vi "tsapp_add_cyclic_msg_can_win32.vi"(8 "错误输入（无错误）":errorcluster, 9 "AAppChannel":i32(ring) items=["CHN1", "CHN2", "CHN3", "CHN4", "CHN5", "CHN6", "CHN7", "CHN8", "CHN9", "CHN10", "CHN11", "CHN12", "CHN13", "CHN14", "CHN15", "CHN16", "CHN17", "CHN18", "CHN19", "CHN20", "CHN21", "CHN22", "CHN23", "CHN24", "CHN25", "CHN26", "CHN27", "CHN28", "CHN29", "CHN30", "CHN31", "CHN32"], 10 "APeriodMS":sgl, 11 "数据帧信息":T1 {"ADLC" max=64; "AID" max=536870911}) -> (0 "错误输出":errorcluster, 3 "tsapp_add_cyclic_msg_can":i32)   [LabVIEW 2016]
uses:
  Ctrl/CAN_FrameInfo.ctl
  TCANProperty.ctl
  SendMsgInfo.ctl
  TSMaster.dll
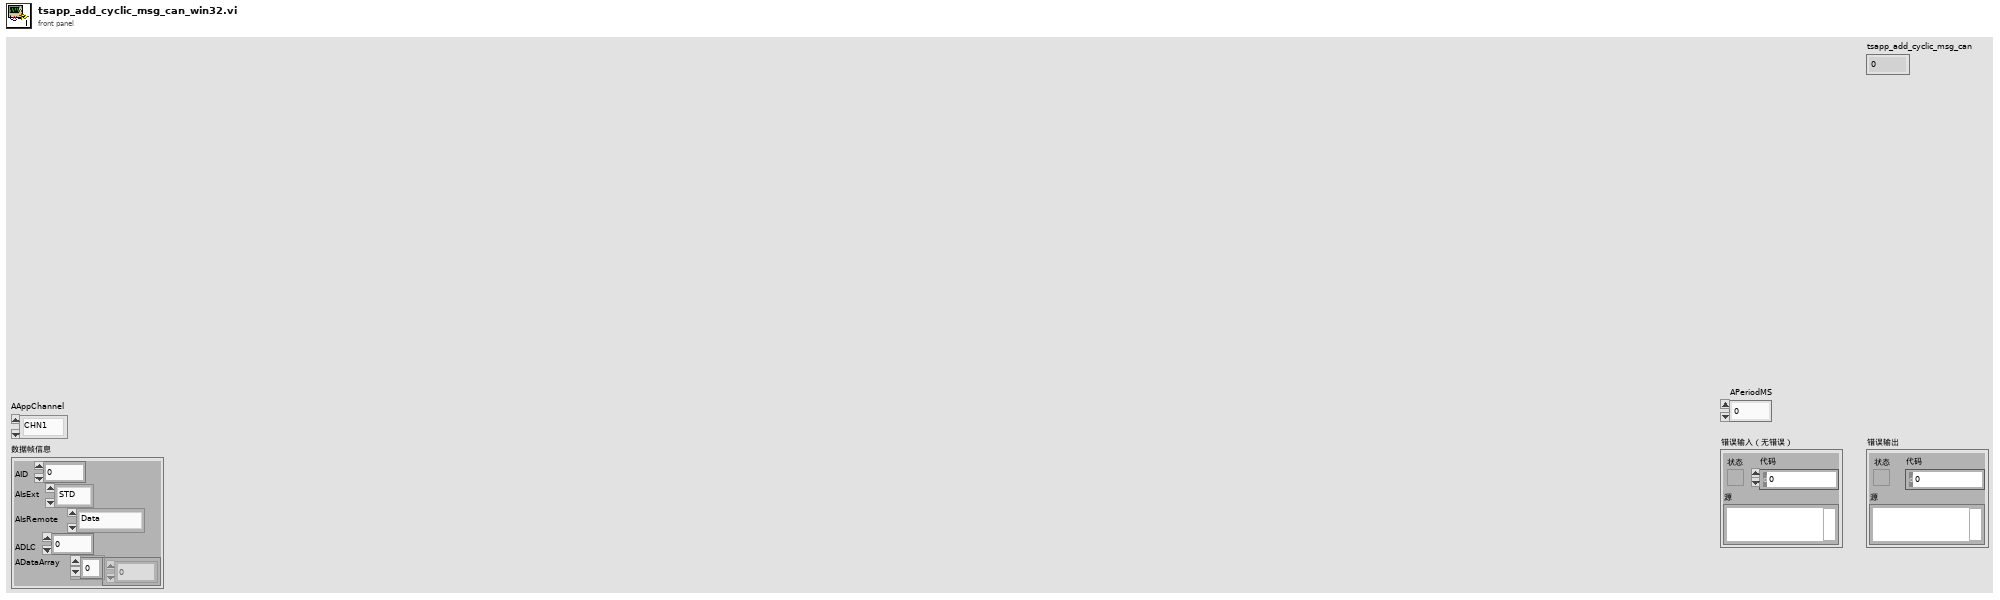
[diagram p1: front panel]
types:
  T1 = typedef "CAN_FrameInfo.ctl" = cluster{"AID":u32, "AIsExt":enum16{"STD", "EXT"}, "AIsRemote":enum16{"Data", "Remote"}, "ADLC":u8, "ADataArray":u8[]}
  T2 = typedef "SendMsgInfo.ctl" = cluster{"FIdxChn":u8, "FProperties":u8, "FDLC":u8, "FReserved":u8, "FIdentifier":i32, "FTimeUS":u64, "Data0":u8, "Data1":u8, "Data2":u8, "Data3":u8, "Data4":u8, "Data5":u8, "Data6":u8, "Data7":u8}
  T3 = typedef "TCANProperty.ctl" = cluster{"istx":bool, "remoteframe":bool, "extframe":bool, "tbd1":bool, "tbd2":bool, "tbd3":bool, "tbd4":bool, "iserrorframe":bool}
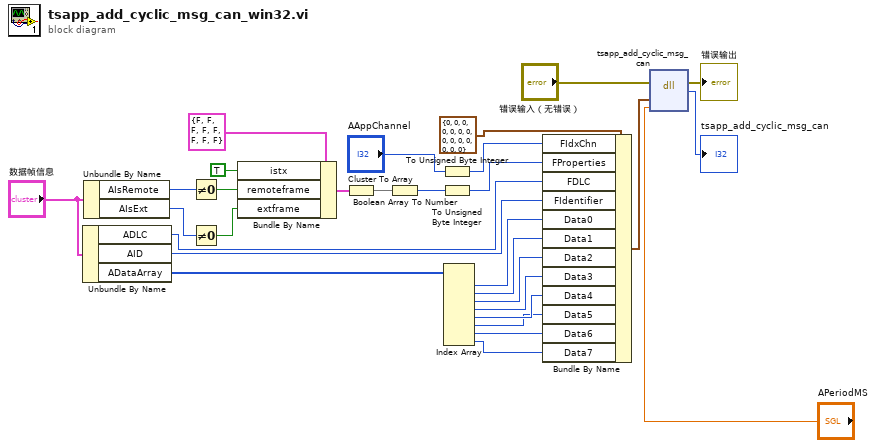
[diagram p0: block diagram]
diagram:
  n1 = Unbundle By Name("数据帧信息") -> ("ADLC"=w12:u8, "AID"=w11:u32, "ADataArray"=w10:u8[])
  n2 = Unbundle By Name("数据帧信息") -> ("AIsRemote"=w19:enum16{"Data", "Remote"}, "AIsExt"=w17:enum16{"STD", "EXT"})
  n3 = Not Equal To 0?(x=w19) -> (x != 0?=w20:bool)
  n4 = Not Equal To 0?(x=w17) -> (x != 0?=w18:bool)
  n5 = Bundle By Name(cluster=T3 {"istx"=FALSE, "remoteframe"=FALSE, "extframe"=FALSE, "tbd1"=FALSE, "tbd2"=FALSE, "tbd3"=FALSE, "tbd4"=FALSE, "iserrorframe"=FALSE} ("TCANProperty"), "istx"=TRUE, "remoteframe"=w20, "extframe"=w18) -> (w16:T3)
  n6 = Cluster To Array(cluster=w16) -> (array=w15:bool[])
  n7 = Boolean Array To Number(Boolean array=w15) -> (number=w14:u32)
  n8 = To Unsigned Byte Integer(number="AAppChannel") -> (unsigned 8bit integer=w23:u8)
  n9 = To Unsigned Byte Integer(number=w14) -> (unsigned 8bit integer=w13:u8)
  n10 = Index Array(array=w10) -> (element #1=w9:u8, element #2=w8:u8, element #3=w7:u8, element #4=w6:u8, element #5=w5:u8, element #6=w4:u8, element #7=w3:u8, element #8=w2:u8)  [unwired: 8 in]
  n11 = Bundle By Name(cluster=T2 {"FIdxChn"=0, "FProperties"=0, "FDLC"=0, "FReserved"=0, "FIdentifier"=0, "FTimeUS"=0, "Data0"=0, "Data1"=0, "Data2"=0, "Data3"=0, "Data4"=0, "Data5"=0, "Data6"=0, "Data7"=0} ("SendMsgInfo"), "FIdxChn"=w23, "FProperties"=w13, "FDLC"=w12, "FIdentifier"=w11, "Data0"=w9, "Data1"=w8, "Data2"=w7, "Data3"=w6, "Data4"=w5, "Data5"=w4, "Data6"=w3, "Data7"=w2) -> (w1:T2)
  n12 = dll-call lib="C:/Users/Eric/Desktop/LabVIEW/TSMasterAPI/Win32/CANopen_TS_2015/TSMaster.dll" fn="tsapp_add_cyclic_msg_can"(error in="错误输入（无错误）", "ACAN"=w1, "APeriodMS"="APeriodMS") -> (error out=→"错误输出":errorcluster, "tsapp_add_cyclic_msg_can"=→"tsapp_add_cyclic_msg_can":i32)  [unwired: 4 in, 1 out]
